vi "MakeXYZAxes.vi"(0 "Field Magnitude":sgl=1.0, 1 "Field Phi":sgl, 2 "Field Theta":sgl, 3 "Target Magnitude":sgl=1.0, 4 "Target Phi":sgl, 5 "Target Theta":sgl, 7 "error in (no error)":errorcluster) -> (9 "error out":errorcluster, 14 "Field Graph":refnum<vi>, 17 "Legend":refnum<vi>)   [LabVIEW 2016]
uses:
  <vilib>/Utility/miscctls.llb/LVSceneTextAlignment.ctl
  <vilib>/picture/3D Picture Control/Object/Create Object (name).vi
  <vilib>/picture/3D Picture Control/Object/Create Object (drawable).vi
  <vilib>/picture/3D Picture Control/Object/Add Object (no reference).vi
  <vilib>/picture/3D Picture Control/NI_3D Picture Control.lvlib
panel:
  in  "Scene Name":string="VRM"
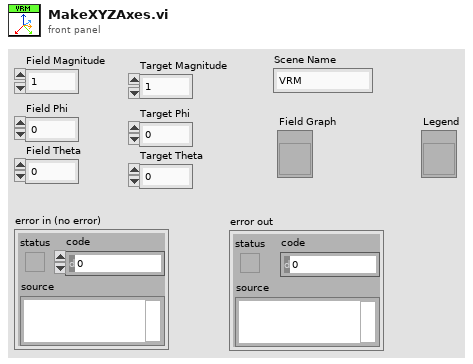
[diagram p1: front panel]
types:
  T1 = typedef "LVSceneTextAlignment.ctl" = cluster{"Horizontal Alignment":enum8{"Left", "Right", "Center"}, "Vertical Alignment":enum8{"Top", "Bottom", "Center", "Base Line", "Bottom Base Line"}}
  T2 = cluster{"Alignment":T1, "Axis Alignment":enum8{"X-Y", "Y-Z", "X-Z", "Reversed X-Y", "Reversed Y-Z", "Reversed X-Z", "Screen"}, "Vertical?":bool, "Wrap Distance":sgl}
  T3 = cluster{"Red":sgl, "Green":sgl, "Blue":sgl, "Alpha":sgl}
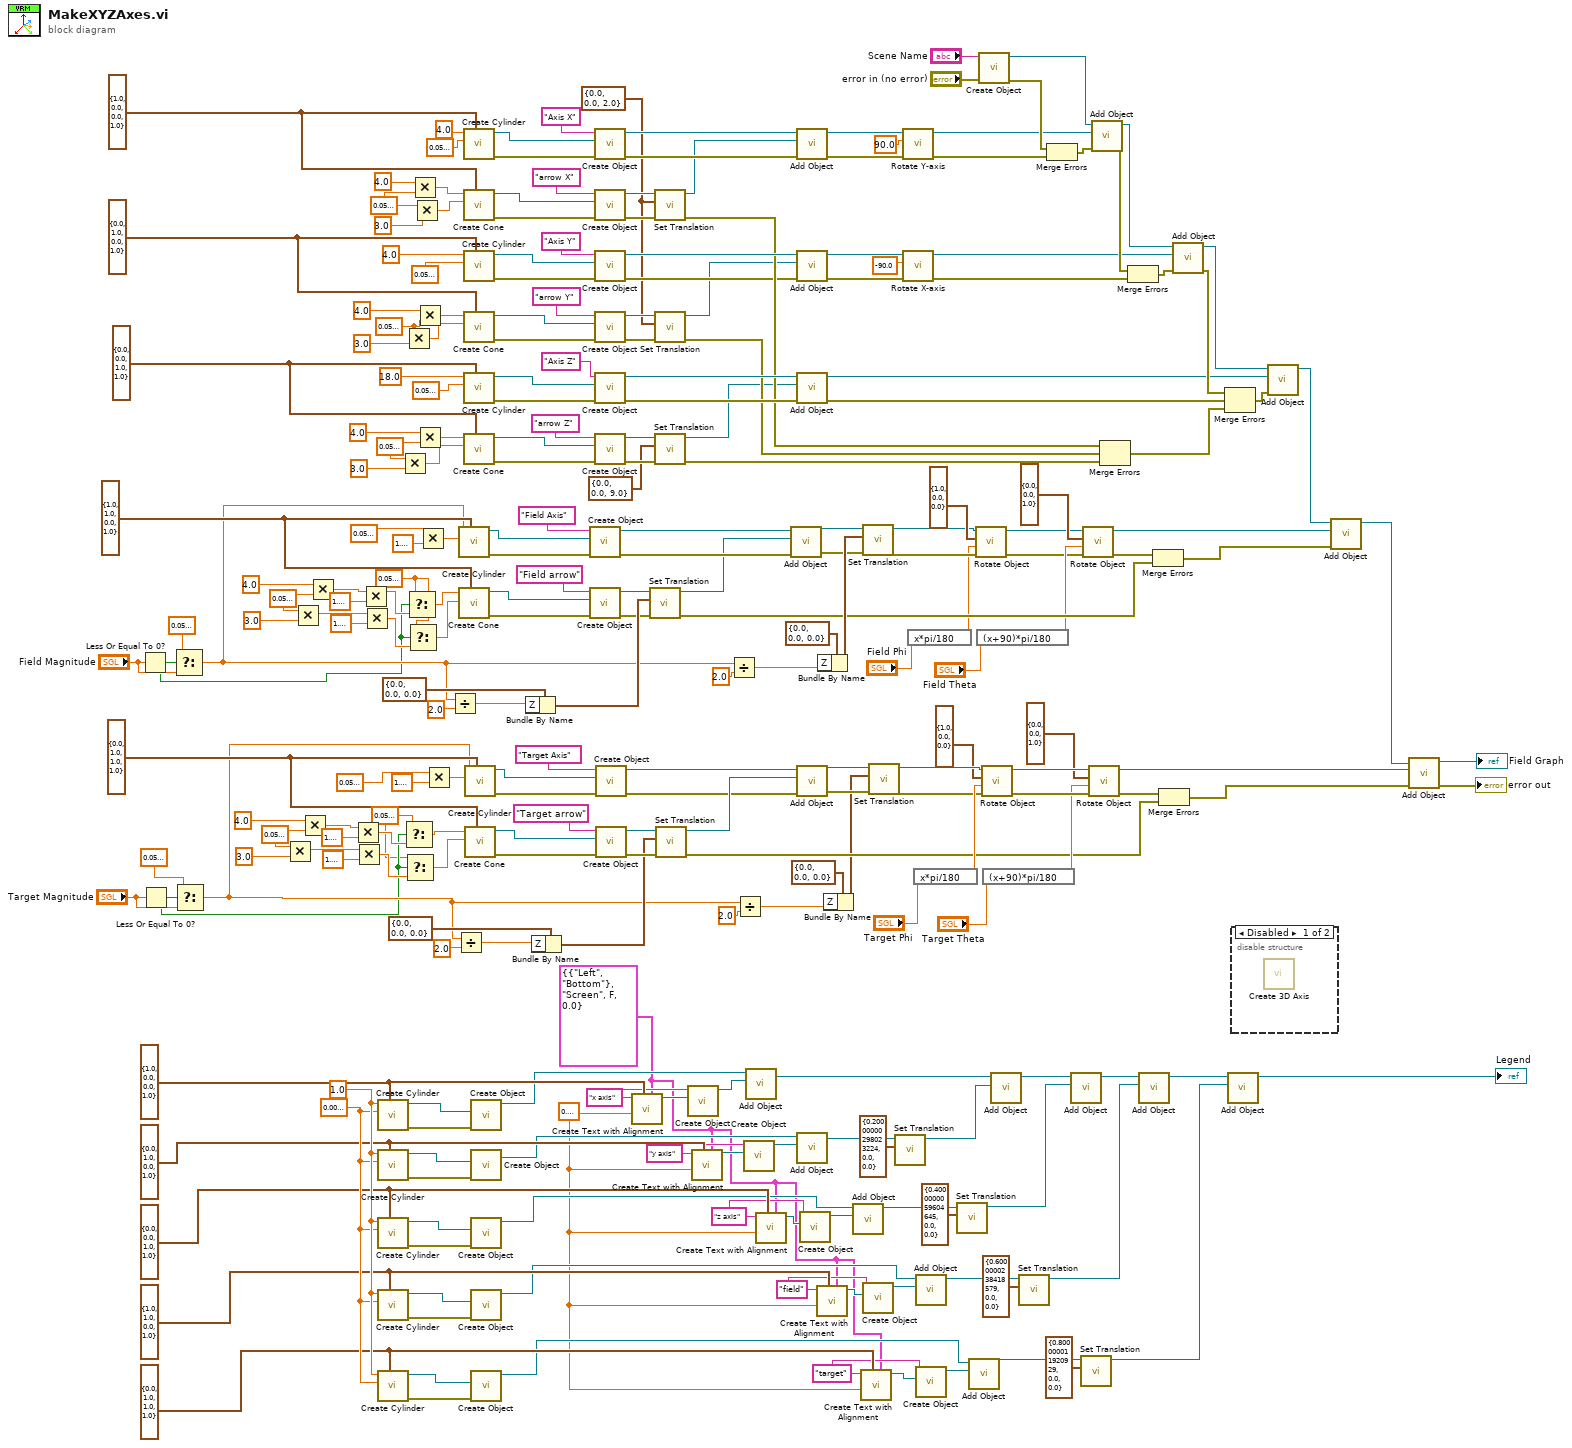
[diagram p0: block diagram]
diagram:
  w2 = sgl 0.2 ("Character Size")
  w3 = T2 {"Alignment"={"Horizontal Alignment"=enum."Left", "Vertical Alignment"=enum."Bottom"}, "Axis Alignment"=enum."Screen", "Vertical?"=FALSE, "Wrap Distance"=0.0} ("Font Options")
  w27 = "target" ("Text")
  w26 = "field" ("Text")
  w25 = "z axis" ("Text")
  w30 = "y axis" ("Text")
  w33 = "x axis" ("Text")
  w39 = T3 {"Red"=1.0, "Green"=1.0, "Blue"=0.0, "Alpha"=1.0} ("Color")
  w55 = sgl 0.01 ("Radius")
  w56 = sgl 1.0 ("Height")
  w40 = T3 {"Red"=0.0, "Green"=1.0, "Blue"=1.0, "Alpha"=1.0} ("Color")
  w37 = T3 {"Red"=1.0, "Green"=0.0, "Blue"=0.0, "Alpha"=1.0} ("Color")
  w36 = T3 {"Red"=0.0, "Green"=0.0, "Blue"=1.0, "Alpha"=1.0} ("Color")
  w38 = T3 {"Red"=0.0, "Green"=1.0, "Blue"=0.0, "Alpha"=1.0} ("Color")
  w59 = sgl 0.05 ("Radius")
  w60 = sgl 0.05 ("Radius")
  w78 = sgl 0.05 ("Radius")
  w89 = sgl 0.05 ("Radius")
  w100 = T3 {"Red"=1.0, "Green"=1.0, "Blue"=0.0, "Alpha"=1.0} ("Color")
  w145 = sgl 0.05 ("Radius")
  w140 = sgl 0.05 ("Radius")
  w143 = sgl 0.05 ("Radius")
  w134 = cluster{"X":sgl, "Y":sgl, "Z":sgl} {"X"=0.0, "Y"=0.0, "Z"=2.0} ("Translation")
  w190 = T3 {"Red"=0.0, "Green"=1.0, "Blue"=1.0, "Alpha"=1.0} ("Color")
  w204 = T3 {"Red"=0.0, "Green"=0.0, "Blue"=1.0, "Alpha"=1.0} ("Color")
  w203 = T3 {"Red"=0.0, "Green"=1.0, "Blue"=0.0, "Alpha"=1.0} ("Color")
  w208 = T3 {"Red"=1.0, "Green"=0.0, "Blue"=0.0, "Alpha"=1.0} ("Color")
  n1 = Less Or Equal To 0?(x="Field Magnitude") -> (x <= 0?=w61:bool)
  n2 = Less Or Equal To 0?(x="Target Magnitude") -> (x <= 0?=w62:bool)
  n3 = Select(t=sgl 0.05 ("f"), s=w61, f="Field Magnitude") -> (s? t:f=w76:sgl)
  n4 = Select(t=sgl 0.05 ("f"), s=w62, f="Target Magnitude") -> (s? t:f=w75:sgl)
  n5 = Multiply(x=w89, y=sgl 3.0) -> (x*y=w85:sgl)
  n6 = Multiply(x=w78, y=sgl 3.0) -> (x*y=w82:sgl)
  n7 = Multiply(x=sgl 4.0 ("Height"), y=w89) -> (x*y=w84:sgl)
  n8 = Multiply(x=sgl 4.0 ("Height"), y=w78) -> (x*y=w83:sgl)
  n9 = Multiply(x=w84, y=sgl 1.1) -> (x*y=w66:sgl)
  n10 = Multiply(x=w85, y=sgl 1.1) -> (x*y=w65:sgl)
  n11 = Multiply(x=w83, y=sgl 1.1) -> (x*y=w70:sgl)
  n12 = Multiply(x=w82, y=sgl 1.1) -> (x*y=w69:sgl)
  n13 = call <vilib>:"Create Cylinder.vi"("Color"=w37, "Radius"=w55, "Height"=w56) -> ("error out"=w54:errorcluster, "New Cylinder Refnum"=w49:refnum<vi>)  [unwired: 7 in]
  n14 = call <vilib>:"Create Cylinder.vi"("Color"=w38, "Radius"=w55, "Height"=w56) -> ("error out"=w53:errorcluster, "New Cylinder Refnum"=w48:refnum<vi>)  [unwired: 7 in]
  n15 = call <vilib>:"Create Cylinder.vi"("Color"=w36, "Radius"=w55, "Height"=w56) -> ("error out"=w52:errorcluster, "New Cylinder Refnum"=w47:refnum<vi>)  [unwired: 7 in]
  n16 = call <vilib>:"Create Cylinder.vi"("Color"=w39, "Radius"=w55, "Height"=w56) -> ("error out"=w51:errorcluster, "New Cylinder Refnum"=w46:refnum<vi>)  [unwired: 7 in]
  n17 = call <vilib>:"Create Cylinder.vi"("Color"=w40, "Radius"=w55, "Height"=w56) -> ("error out"=w50:errorcluster, "New Cylinder Refnum"=w45:refnum<vi>)  [unwired: 7 in]
  n18 = Multiply(x=w145, y=sgl 3.0) -> (x*y=w146:sgl)
  n19 = Multiply(x=w140, y=sgl 3.0) -> (x*y=w153:sgl)
  n20 = Select(t=w59, s=w62, f=w66) -> (s? t:f=w63:sgl)
  n21 = Select(t=w59, s=w62, f=w65) -> (s? t:f=w64:sgl)
  n22 = Select(t=w60, s=w61, f=w70) -> (s? t:f=w67:sgl)
  n23 = Select(t=w60, s=w61, f=w69) -> (s? t:f=w68:sgl)
  n24 = Multiply(x=sgl 4.0 ("Height"), y=w143) -> (x*y=w141:sgl)
  n25 = Multiply(x=w143, y=sgl 3.0) -> (x*y=w160:sgl)
  n26 = Multiply(x=sgl 4.0 ("Height"), y=w140) -> (x*y=w151:sgl)
  n27 = Multiply(x=sgl 4.0 ("Height"), y=w145) -> (x*y=w148:sgl)
  n28 = Multiply(x=sgl 0.05 ("y"), y=sgl 1.1) -> (x*y=w126:sgl)
  n29 = Multiply(x=sgl 0.05 ("y"), y=sgl 1.1) -> (x*y=w162:sgl)
  n30 = Divide(x=w76, y=sgl 2.0 ("x")) -> (x/y=w107:sgl)
  n31 = Divide(x=w75, y=sgl 2.0 ("x")) -> (x/y=w181:sgl)
  n32 = call <vilib>:"Create Cylinder.vi"("Color"=w100, "Radius"=w126, "Height"=w76) -> ("error out"=w99:errorcluster, "New Cylinder Refnum"=w112:refnum<vi>)  [unwired: 7 in]
  n33 = call <vilib>:"Create Cone.vi"("Color"=w100, "Radius"=w68, "Height"=w67) -> ("error out"=w93:errorcluster, "New Cone Refnum"=w111:refnum<vi>)  [unwired: 7 in]
  n34 = call <vilib>:"Create Cylinder.vi"("Color"=w208, "Radius"=sgl 0.05, "Height"=sgl 4.0) -> ("error out"=w245:errorcluster, "New Cylinder Refnum"=w248:refnum<vi>)  [unwired: 7 in]
  n35 = call <vilib>:"Create Cone.vi"("Color"=w208, "Radius"=w160, "Height"=w141) -> ("error out"=w209:errorcluster, "New Cone Refnum"=w225:refnum<vi>)  [unwired: 7 in]
  n36 = call <vilib>:"Create Cylinder.vi"("Color"=w203, "Radius"=sgl 0.05, "Height"=sgl 4.0) -> ("error out"=w244:errorcluster, "New Cylinder Refnum"=w250:refnum<vi>)  [unwired: 7 in]
  n37 = call <vilib>:"Create Cone.vi"("Color"=w203, "Radius"=w153, "Height"=w151) -> ("error out"=w205:errorcluster, "New Cone Refnum"=w199:refnum<vi>)  [unwired: 7 in]
  n38 = call <vilib>:"Create Cylinder.vi"("Color"=w204, "Radius"=sgl 0.05, "Height"=sgl 18.0) -> ("error out"=w243:errorcluster, "New Cylinder Refnum"=w249:refnum<vi>)  [unwired: 7 in]
  n39 = call <vilib>:"Create Cone.vi"("Color"=w204, "Radius"=w146, "Height"=w148) -> ("error out"=w206:errorcluster, "New Cone Refnum"=w207:refnum<vi>)  [unwired: 7 in]
  n40 = call <vilib>:"Create Cylinder.vi"("Color"=w190, "Radius"=w162, "Height"=w75) -> ("error out"=w191:errorcluster, "New Cylinder Refnum"=w176:refnum<vi>)  [unwired: 7 in]
  n41 = call <vilib>:"Create Cone.vi"("Color"=w190, "Radius"=w64, "Height"=w63) -> ("error out"=w197:errorcluster, "New Cone Refnum"=w177:refnum<vi>)  [unwired: 7 in]
  n42 = call-poly <vilib>:"Create Object.vi"("error in (no error)"=w54, "Geometry"=w49) -> ("Scene:New Object"=w35:refnum<vi>)  [unwired: 8 in, 1 out]
  n43 = call-poly <vilib>:"Create Object.vi"("error in (no error)"=w53, "Geometry"=w48) -> ("Scene:New Object"=w28:refnum<vi>)  [unwired: 8 in, 1 out]
  n44 = call-poly <vilib>:"Create Object.vi"("error in (no error)"=w52, "Geometry"=w47) -> ("Scene:New Object"=w20:refnum<vi>)  [unwired: 8 in, 1 out]
  n45 = call-poly <vilib>:"Create Object.vi"("error in (no error)"=w51, "Geometry"=w46) -> ("Scene:New Object"=w18:refnum<vi>)  [unwired: 8 in, 1 out]
  n46 = call-poly <vilib>:"Create Object.vi"("error in (no error)"=w50, "Geometry"=w45) -> ("Scene:New Object"=w16:refnum<vi>)  [unwired: 8 in, 1 out]
  n47 = Bundle By Name(cluster=cluster{"X":sgl, "Y":sgl, "Z":sgl} {"X"=0.0, "Y"=0.0, "Z"=0.0} ("Translation"), "Z"=w107) -> (w110:cluster{"X":sgl, "Y":sgl, "Z":sgl})
  n48 = Bundle By Name(cluster=cluster{"X":sgl, "Y":sgl, "Z":sgl} {"X"=0.0, "Y"=0.0, "Z"=0.0} ("Translation"), "Z"=w181) -> (w178:cluster{"X":sgl, "Y":sgl, "Z":sgl})
  n49 = call-poly <vilib>:"Create Object.vi"("error in (no error)"=w99, "Geometry"=w112, "Name"="Field Axis") -> ("error out"=w95:errorcluster, "Scene:New Object"=w96:refnum<vi>)  [unwired: 7 in]
  n50 = call-poly <vilib>:"Create Object.vi"("error in (no error)"=w93, "Geometry"=w111, "Name"="Field arrow") -> ("error out"=w97:errorcluster, "Scene:New Object"=w98:refnum<vi>)  [unwired: 7 in]
  n51 = call-poly <vilib>:"Create Object.vi"("error in (no error)"=w245, "Geometry"=w248, "Name"="Axis X") -> ("error out"=w218:errorcluster, "Scene:New Object"=w233:refnum<vi>)  [unwired: 7 in]
  n52 = call-poly <vilib>:"Create Object.vi"("error in (no error)"=w209, "Geometry"=w225, "Name"="arrow X") -> ("error out"=w235:errorcluster, "Scene:New Object"=w236:refnum<vi>)  [unwired: 7 in]
  n53 = call-poly <vilib>:"Create Object.vi"("error in (no error)"=w244, "Geometry"=w250, "Name"="Axis Y") -> ("error out"=w211:errorcluster, "Scene:New Object"=w229:refnum<vi>)  [unwired: 7 in]
  n54 = call-poly <vilib>:"Create Object.vi"("error in (no error)"=w205, "Geometry"=w199, "Name"="arrow Y") -> ("error out"=w231:errorcluster, "Scene:New Object"=w230:refnum<vi>)  [unwired: 7 in]
  n55 = call-poly <vilib>:"Create Object.vi"("error in (no error)"=w243, "Geometry"=w249, "Name"="Axis Z") -> ("error out"=w221:errorcluster, "Scene:New Object"=w224:refnum<vi>)  [unwired: 7 in]
  n56 = call-poly <vilib>:"Create Object.vi"("error in (no error)"=w206, "Geometry"=w207, "Name"="arrow Z") -> ("error out"=w226:errorcluster, "Scene:New Object"=w227:refnum<vi>)  [unwired: 7 in]
  n57 = call-poly <vilib>:"Create Object.vi"("error in (no error)"=w191, "Geometry"=w176, "Name"="Target Axis") -> ("error out"=w195:errorcluster, "Scene:New Object"=w194:refnum<vi>)  [unwired: 7 in]
  n58 = call-poly <vilib>:"Create Object.vi"("error in (no error)"=w197, "Geometry"=w177, "Name"="Target arrow") -> ("error out"=w193:errorcluster, "Scene:New Object"=w192:refnum<vi>)  [unwired: 7 in]
  n59 = call <vilib>:"Create Text with Alignment.vi"("Font Options"=w3, "Color"=w37, "Character Size"=w2, "Text"=w33) -> ("New Text Refnum"=w34:refnum<vi>)  [unwired: 6 in, 1 out]
  n60 = call <vilib>:"Set Translation.vi"("error in (no error)"=w97, "Translation"=w110, "Scene Object"=w98) -> ("error out"=w106:errorcluster, "Translated Object"=w92:refnum<vi>)  [unwired: 7 in]
  n61 = call <vilib>:"Set Translation.vi"("error in (no error)"=w235, "Translation"=w134, "Scene Object"=w236) -> ("error out"=w215:errorcluster, "Translated Object"=w202:refnum<vi>)  [unwired: 7 in]
  n62 = call <vilib>:"Set Translation.vi"("error in (no error)"=w231, "Translation"=w134, "Scene Object"=w230) -> ("error out"=w214:errorcluster, "Translated Object"=w201:refnum<vi>)  [unwired: 7 in]
  n63 = call <vilib>:"Set Translation.vi"("error in (no error)"=w226, "Translation"=cluster{"X":sgl, "Y":sgl, "Z":sgl} {"X"=0.0, "Y"=0.0, "Z"=9.0}, "Scene Object"=w227) -> ("error out"=w213:errorcluster, "Translated Object"=w200:refnum<vi>)  [unwired: 7 in]
  n64 = call <vilib>:"Set Translation.vi"("error in (no error)"=w193, "Translation"=w178, "Scene Object"=w192) -> ("error out"=w182:errorcluster, "Translated Object"=w198:refnum<vi>)  [unwired: 7 in]
  n65 = call-poly <vilib>:"Create Object.vi"("Geometry"=w34, "Name"=w33) -> ("Scene:New Object"=w32:refnum<vi>)  [unwired: 8 in, 1 out]
  n66 = call <vilib>:"Create Text with Alignment.vi"("Font Options"=w3, "Color"=w38, "Character Size"=w2, "Text"=w30) -> ("New Text Refnum"=w31:refnum<vi>)  [unwired: 6 in, 1 out]
  n67 = Divide(x=w76, y=sgl 2.0) -> (x/y=w121:sgl)
  n68 = Divide(x=w75, y=sgl 2.0) -> (x/y=w167:sgl)
  n69 = call-poly <vilib>:"Create Object.vi"("Geometry"=w31, "Name"=w30) -> ("Scene:New Object"=w29:refnum<vi>)  [unwired: 8 in, 1 out]
  n70 = call-poly <vilib>:"Add Object.vi"("New Object In"=w32, "Scene Object In"=w35) -> ("Scene Object Out"=w11:refnum<vi>)  [unwired: 8 in, 1 out]
  n71 = call <vilib>:"Create Text with Alignment.vi"("Font Options"=w3, "Color"=w36, "Character Size"=w2, "Text"=w25) -> ("New Text Refnum"=w24:refnum<vi>)  [unwired: 6 in, 1 out]
  n72 = call-poly <vilib>:"Add Object.vi"("error in (no error)"=w95, "New Object In"=w92, "Scene Object In"=w96) -> ("error out"=w114:errorcluster, "Scene Object Out"=w115:refnum<vi>)  [unwired: 7 in]
  n73 = call-poly <vilib>:"Add Object.vi"("error in (no error)"=w218, "New Object In"=w202, "Scene Object In"=w233) -> ("error out"=w217:errorcluster, "Scene Object Out"=w232:refnum<vi>)  [unwired: 7 in]
  n74 = call-poly <vilib>:"Add Object.vi"("error in (no error)"=w211, "New Object In"=w201, "Scene Object In"=w229) -> ("error out"=w210:errorcluster, "Scene Object Out"=w228:refnum<vi>)  [unwired: 7 in]
  n75 = call-poly <vilib>:"Add Object.vi"("error in (no error)"=w221, "New Object In"=w200, "Scene Object In"=w224) -> ("error out"=w220:errorcluster, "Scene Object Out"=w222:refnum<vi>)  [unwired: 7 in]
  n76 = call-poly <vilib>:"Add Object.vi"("error in (no error)"=w195, "New Object In"=w198, "Scene Object In"=w194) -> ("error out"=w174:errorcluster, "Scene Object Out"=w173:refnum<vi>)  [unwired: 7 in]
  n77 = call-poly <vilib>:"Add Object.vi"("New Object In"=w29, "Scene Object In"=w28) -> ("Scene Object Out"=w12:refnum<vi>)  [unwired: 8 in, 1 out]
  n78 = call-poly <vilib>:"Create Object.vi"("Geometry"=w24, "Name"=w25) -> ("Scene:New Object"=w21:refnum<vi>)  [unwired: 8 in, 1 out]
  n79 = call <vilib>:"Create Text with Alignment.vi"("Font Options"=w3, "Color"=w39, "Character Size"=w2, "Text"=w26) -> ("New Text Refnum"=w23:refnum<vi>)  [unwired: 6 in, 1 out]
  n80 = Bundle By Name(cluster=cluster{"X":sgl, "Y":sgl, "Z":sgl} {"X"=0.0, "Y"=0.0, "Z"=0.0} ("Translation"), "Z"=w121) -> (w119:cluster{"X":sgl, "Y":sgl, "Z":sgl})
  n81 = Bundle By Name(cluster=cluster{"X":sgl, "Y":sgl, "Z":sgl} {"X"=0.0, "Y"=0.0, "Z"=0.0} ("Translation"), "Z"=w167) -> (w169:cluster{"X":sgl, "Y":sgl, "Z":sgl})
  n82 = call-poly <vilib>:"Add Object.vi"("New Object In"=w21, "Scene Object In"=w20) -> ("Scene Object Out"=w13:refnum<vi>)  [unwired: 8 in, 1 out]
  n83 = call <vilib>:"Create Text with Alignment.vi"("Font Options"=w3, "Color"=w40, "Character Size"=w2, "Text"=w27) -> ("New Text Refnum"=w22:refnum<vi>)  [unwired: 6 in, 1 out]
  n84 = call <vilib>:"Set Translation.vi"("error in (no error)"=w114, "Translation"=w119, "Scene Object"=w115) -> ("error out"=w117:errorcluster, "Translated Object"=w116:refnum<vi>)  [unwired: 7 in]
  n85 = call-poly <vilib>:"Create Object.vi"("Geometry"=w23, "Name"=w26) -> ("Scene:New Object"=w19:refnum<vi>)  [unwired: 8 in, 1 out]
  n86 = call <vilib>:"Set Translation.vi"("error in (no error)"=w174, "Translation"=w169, "Scene Object"=w173) -> ("error out"=w171:errorcluster, "Translated Object"=w172:refnum<vi>)  [unwired: 7 in]
  n87 = call <vilib>:"Set Translation.vi"("Translation"=cluster{"X":sgl, "Y":sgl, "Z":sgl} {"X"=0.2, "Y"=0.0, "Z"=0.0}, "Scene Object"=w12) -> ("Translated Object"=w10:refnum<vi>)  [unwired: 8 in, 1 out]
  n88 = call <vilib>:"Rotate Y-axis.vi"("error in (no error)"=w217, "angle"=90.0, "Scene Object In"=w232) -> ("error out"=w216:errorcluster, "Scene Object Out"=w234:refnum<vi>)  [unwired: 7 in]
  n89 = call <vilib>:"Rotate X-axis.vi"("error in (no error)"=w210, "angle"=-90.0, "Scene Object In"=w228) -> ("error out"=w219:errorcluster, "Scene Object Out"=w223:refnum<vi>)  [unwired: 7 in]
  n90 = expression code="x*pi/180"("Field Phi") -> (w104:sgl)
  n91 = expression code="x*pi/180"("Target Phi") -> (w186:sgl)
  n92 = call-poly <vilib>:"Add Object.vi"("New Object In"=w19, "Scene Object In"=w18) -> ("Scene Object Out"=w14:refnum<vi>)  [unwired: 8 in, 1 out]
  n93 = call-poly <vilib>:"Create Object.vi"("Geometry"=w22, "Name"=w27) -> ("Scene:New Object"=w17:refnum<vi>)  [unwired: 8 in, 1 out]
  n94 = call <vilib>:"Set Translation.vi"("Translation"=cluster{"X":sgl, "Y":sgl, "Z":sgl} {"X"=0.4, "Y"=0.0, "Z"=0.0}, "Scene Object"=w13) -> ("Translated Object"=w9:refnum<vi>)  [unwired: 8 in, 1 out]
  n95 = call-poly <vilib>:"Add Object.vi"("New Object In"=w17, "Scene Object In"=w16) -> ("Scene Object Out"=w15:refnum<vi>)  [unwired: 8 in, 1 out]
  n96 = call <vilib>:"Rotate Object.vi"("error in (no error)"=w117, "Angle"=w104, "Axis"=cluster{"X":sgl, "Y":sgl, "Z":sgl} {"X"=1.0, "Y"=0.0, "Z"=0.0}, "Scene.Object In"=w116) -> ("error out"=w102:errorcluster, "Scene.Object Out"=w101:refnum<vi>)  [unwired: 6 in]
  n97 = expression code="(x+90)*pi/180"("Field Theta") -> (w103:sgl)
  n98 = call-poly <vilib>:"Create Object.vi"("error in (no error)"="error in (no error)", "Name"="Scene Name") -> ("error out"=w242:errorcluster, "Scene:New Object"=w255:refnum<vi>)  [unwired: 8 in]
  n99 = call <vilib>:"Rotate Object.vi"("error in (no error)"=w171, "Angle"=w186, "Axis"=cluster{"X":sgl, "Y":sgl, "Z":sgl} {"X"=1.0, "Y"=0.0, "Z"=0.0}, "Scene.Object In"=w172) -> ("error out"=w188:errorcluster, "Scene.Object Out"=w189:refnum<vi>)  [unwired: 6 in]
  n100 = expression code="(x+90)*pi/180"("Target Theta") -> (w187:sgl)
  n101 = call-poly <vilib>:"Add Object.vi"("New Object In"=w10, "Scene Object In"=w11) -> ("Scene Object Out"=w8:refnum<vi>)  [unwired: 8 in, 1 out]
  n102 = call <vilib>:"Set Translation.vi"("Translation"=cluster{"X":sgl, "Y":sgl, "Z":sgl} {"X"=0.6, "Y"=0.0, "Z"=0.0}, "Scene Object"=w14) -> ("Translated Object"=w7:refnum<vi>)  [unwired: 8 in, 1 out]
  n103 = Merge Errors(w242, w216) -> (w241:errorcluster)
  n104 = call-poly <vilib>:"Add Object.vi"("New Object In"=w9, "Scene Object In"=w8) -> ("Scene Object Out"=w6:refnum<vi>)  [unwired: 8 in, 1 out]
  n105 = call <vilib>:"Set Translation.vi"("Translation"=cluster{"X":sgl, "Y":sgl, "Z":sgl} {"X"=0.8, "Y"=0.0, "Z"=0.0}, "Scene Object"=w15) -> ("Translated Object"=w5:refnum<vi>)  [unwired: 8 in, 1 out]
  n106 = call <vilib>:"Rotate Object.vi"("error in (no error)"=w102, "Angle"=w103, "Axis"=cluster{"X":sgl, "Y":sgl, "Z":sgl} {"X"=0.0, "Y"=0.0, "Z"=1.0}, "Scene.Object In"=w101) -> ("error out"=w122:errorcluster, "Scene.Object Out"=w123:refnum<vi>)  [unwired: 6 in]
  n107 = call <vilib>:"Rotate Object.vi"("error in (no error)"=w188, "Angle"=w187, "Axis"=cluster{"X":sgl, "Y":sgl, "Z":sgl} {"X"=0.0, "Y"=0.0, "Z"=1.0}, "Scene.Object In"=w189) -> ("error out"=w166:errorcluster, "Scene.Object Out"=w165:refnum<vi>)  [unwired: 6 in]
  n108 = call-poly <vilib>:"Add Object.vi"("error in (no error)"=w241, "New Object In"=w234, "Scene Object In"=w255) -> ("error out"=w240:errorcluster, "Scene Object Out"=w254:refnum<vi>)  [unwired: 7 in]
  n109 = Merge Errors(w215, w214, w213) -> (w212:errorcluster)
  n110 = Merge Errors(w240, w219) -> (w239:errorcluster)
  n111 = call-poly <vilib>:"Add Object.vi"("New Object In"=w7, "Scene Object In"=w6) -> ("Scene Object Out"=w4:refnum<vi>)  [unwired: 8 in, 1 out]
  n112 = Merge Errors(w122, w106) -> (w105:errorcluster)
  n113 = Merge Errors(w166, w182) -> (w185:errorcluster)
  n114 = call-poly <vilib>:"Add Object.vi"("error in (no error)"=w239, "New Object In"=w223, "Scene Object In"=w254) -> ("error out"=w238:errorcluster, "Scene Object Out"=w253:refnum<vi>)  [unwired: 7 in]
  n115 = Merge Errors(w238, w220, w212) -> (w237:errorcluster)
  n116 = call-poly <vilib>:"Add Object.vi"("New Object In"=w5, "Scene Object In"=w4) -> ("Scene Object Out"=→"Legend":refnum<vi>)  [unwired: 8 in, 1 out]
  n117 = disable-structure shown="Disabled" {
    frame Disabled {
      n118 = call <vilib>:"Create 3D Axis.vi"() -> ()  [unwired: 10 in, 2 out]
    }
    frame Enabled {
    }
  }
  n119 = call-poly <vilib>:"Add Object.vi"("error in (no error)"=w237, "New Object In"=w222, "Scene Object In"=w253) -> ("Scene Object Out"=w91:refnum<vi>)  [unwired: 7 in, 1 out]
  n120 = call-poly <vilib>:"Add Object.vi"("error in (no error)"=w105, "New Object In"=w123, "Scene Object In"=w91) -> ("Scene Object Out"=w90:refnum<vi>)  [unwired: 7 in, 1 out]
  n121 = call-poly <vilib>:"Add Object.vi"("error in (no error)"=w185, "New Object In"=w165, "Scene Object In"=w90) -> ("error out"=→"error out":errorcluster, "Scene Object Out"=→"Field Graph":refnum<vi>)  [unwired: 7 in]
